vi "Queue Driver with varient.vi"(0 "Name":string, 5 "State In":T1, 7 "N State In":T1[](array[typedef]), 11 "Error In":errorcluster, 13 "Mode":T2) -> (4 "State Out":T1, 6 "Remaining States":T1[](array[typedef]), 15 "Error Out":errorcluster)   [LabVIEW 2020, in "Producer&Consumer - Washing Machine.lvlib"]
doc: "This VI is a LV2, which is used to create Queue driver."
uses:
  Producer&Consumer - Washing Machine.lvlib
  Queue Driver with varient mode.ctl
  Queue Driver with varient mode - N State In.ctl
  String based State machine - Airplane.lvlib
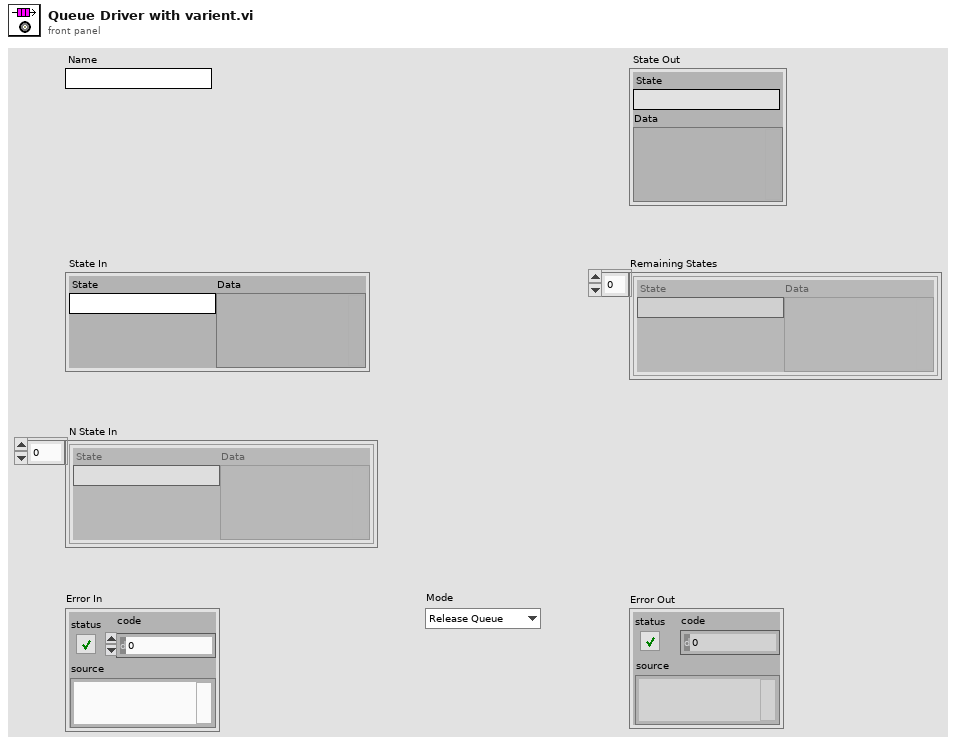
[diagram p1: front panel]
types:
  T1 = typedef "String based State machine - Airplane.lvlib/Queue Driver with varient mode - N State In.ctl" = cluster{"State ":string, "Data":variant}
  T2 = typedef "Producer&Consumer - Washing Machine.lvlib/Queue Driver with varient mode.ctl" = enum16{"Release Queue", "Enstack", "Flush Queue", "Enqueue N", "Dequeue", "Enqueue", "Create Queue"}
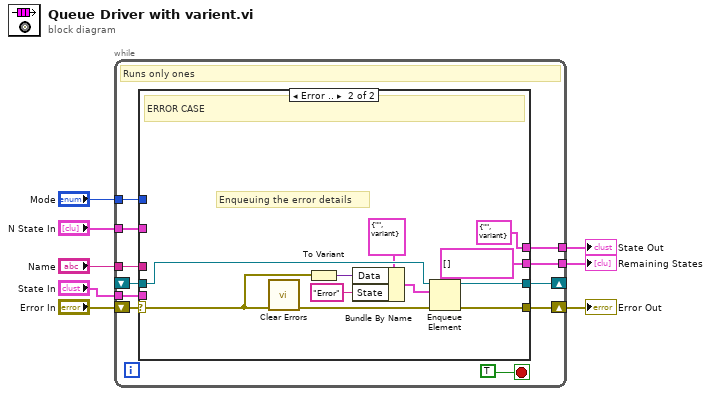
[diagram p0: block diagram]
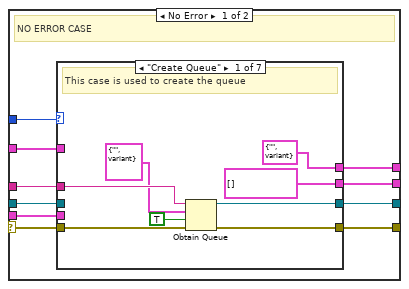
[diagram p2: hidden frame]
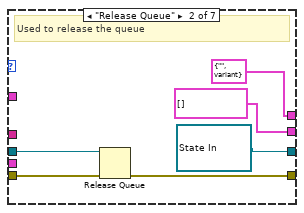
[diagram p3: hidden frame]
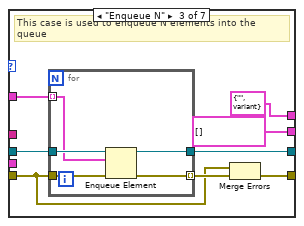
[diagram p4: hidden frame]
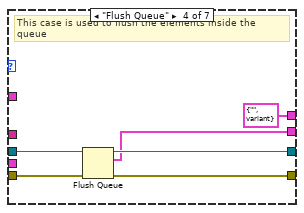
[diagram p5: hidden frame]
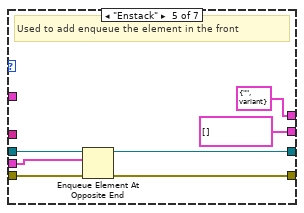
[diagram p6: hidden frame]
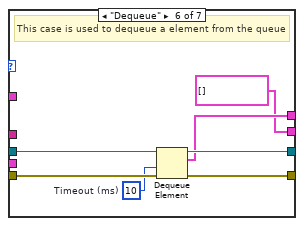
[diagram p7: hidden frame]
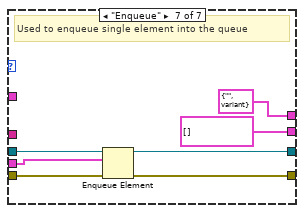
[diagram p8: hidden frame]
diagram:
  n1 = while {
    tunnel: "Mode" -> [w17]
    shift-right: [w18] -> w7
    shift-left: "Error In" -> [w19]
    tunnel: "Name" -> [w16]
    tunnel: [w15] -> w2
    shift-right: [w13] -> _
    shift-left: _ -> [w14]
    tunnel: "N State In" -> [w11]
    tunnel: "State In" -> [w10]
    tunnel: [w9] -> w1
    stop <- TRUE stop-if-true
    # "Runs only ones"
    n2 = case shown="Error .." w19 {
      selector: w19 -> [w28 w88]
      tunnel: [w29 w93] -> w18
      tunnel: w17 -> [w23 _]
      tunnel: w16 -> [w27 _]
      tunnel: [w26 T1 {"State "="", "Data"=variant} ("State In")] -> w15
      tunnel: w14 -> [w25 w92]
      tunnel: [w24 w91] -> w13
      tunnel: w11 -> [w22 _]
      tunnel: w10 -> [w21 _]
      tunnel: [w20 T1[] [] ("remaining elements")] -> w9
      frame No Error {
        # "NO ERROR CASE"
        n3 = case shown="\"Create Queue\"" w23 {
          tunnel: [w37 w43 w47 w62 w69 w76 w83] -> w29
          tunnel: w28 -> [w36 w42 w46 w61 w68 w75 w82]
          tunnel: w27 -> [w35 _ _ _ _ _ _]
          tunnel: [w33 refnum<queue> refnum ("queue out") w49 w59 w66 w73 w80] -> w24
          tunnel: w25 -> [_ w40 w50 w60 w67 w74 w81]
          tunnel: [T1 {"State "="", "Data"=variant} ("State In") T1 {"State "="", "Data"=variant} ("State In") T1 {"State "="", "Data"=variant} ("State In") T1 {"State "="", "Data"=variant} ("State In") T1 {"State "="", "Data"=variant} ("State In") w72 T1 {"State "="", "Data"=variant} ("State In")] -> w26
          tunnel: w22 -> [_ _ w48 _ _ _ _]
          tunnel: w21 -> [_ _ _ _ w65 _ w79]
          tunnel: [T1[] [] ("remaining elements") T1[] [] ("remaining elements") T1[] [] ("remaining elements") w58 T1[] [] ("remaining elements") T1[] [] ("remaining elements") T1[] [] ("remaining elements")] -> w20
          frame "Create Queue" {
            # "This case is used to create the queue"
            n4 = Obtain Queue(name (unnamed)=w35, element data type=T1 {"State "="", "Data"=variant} ("State In"), create if not found? (T)=TRUE, error in (no error)=w36) -> (queue out=w33:refnum<queue>, error out=w37:errorcluster)  [unwired: 1 in, 1 out]
          }
          frame "Release Queue" {
            # "Used to release the queue"
            n5 = Release Queue(queue=w40, error in (no error)=w42) -> (error out=w43:errorcluster)  [unwired: 1 in, 2 out]
          }
          frame "Enqueue N" {
            # "This case is used to enqueue N elements into the queue"
            n6 = for {
              tunnel: w50 -> [w54]
              tunnel: [w53] -> w49
              tunnel: w48 -> [w52] mode=indexing
              tunnel: w46 -> [w55]
              tunnel: [w56] -> w51 mode=indexing
              n7 = Enqueue Element(queue=w54, element=w52, error in (no error)=w55) -> (queue out=w53:refnum<queue>, error out=w56:errorcluster)  [unwired: 1 in, 1 out]
            }
            n8 = Merge Errors(w46, w51) -> (w47:errorcluster)
          }
          frame "Flush Queue" {
            # "This case is used to flush the elements inside the queue"
            n9 = Flush Queue(queue=w60, error in (no error)=w61) -> (queue out=w59:refnum<queue>, remaining elements=w58:T1[], error out=w62:errorcluster)
          }
          frame "Enstack" {
            # "Used to add enqueue the element in the front"
            n10 = Enqueue Element At Opposite End(queue=w67, element=w65, error in (no error)=w68) -> (queue out=w66:refnum<queue>, error out=w69:errorcluster)  [unwired: 1 in, 1 out]
          }
          frame "Dequeue" {
            w71 = 10  # Timeout (ms)
            # "This case is used to dequeue a element from the queue"
            n11 = Dequeue Element(queue=w74, timeout in ms (-1)=w71, error in (no error)=w75) -> (queue out=w73:refnum<queue>, element=w72:T1, error out=w76:errorcluster)  [unwired: 1 out]
          }
          frame "Enqueue" {
            # "Used to enqueue single element into the queue"
            n12 = Enqueue Element(queue=w81, element=w79, error in (no error)=w82) -> (queue out=w80:refnum<queue>, error out=w83:errorcluster)  [unwired: 1 in, 1 out]
          }
        }
      }
      frame Error {
        # "Enqueuing the error details"
        # "ERROR CASE"
        n13 = call <vilib>:"Clear Errors.vi"("error in (no error)"=w88) -> ("error out"=w94:errorcluster)  [unwired: 5 in, 1 out]
        n14 = To Variant(anything=w88) -> (Variant=w87:variant)
        n15 = Bundle By Name(cluster=T1 {"State "="", "Data"=variant} ("element"), "Data"=w87, "State"="Error") -> (w90:T1)
        n16 = Enqueue Element(queue=w92, element=w90, error in (no error)=w94) -> (queue out=w91:refnum<queue>, error out=w93:errorcluster)  [unwired: 1 in, 1 out]
      }
    }
  }
  "Error Out" <- w7
  "State Out" <- w2
  "Remaining States" <- w1
